vi "SEEK_Common_Socket_Cmd_Sub_VI.vi"(4 "Time Delay":dbl=10.0, 6 "Common Socket Error in":errorcluster, 7 "Response ID 1":u8, 8 "Operation Message Length 1":i32, 9 "Operation Message ID 1":i32, 11 "connection ID":refnum<k5>) -> (0 "Status":string="Horn Scan Success", 1 "error out":errorcluster, 3 "connection ID":refnum<k5>)   [LabVIEW 2017]
panel:
  out "Response from SC":string
  out "Response from SC":u8
  out "Data written to SC":i32
  # "INPUT"
  # "OUTPUT"
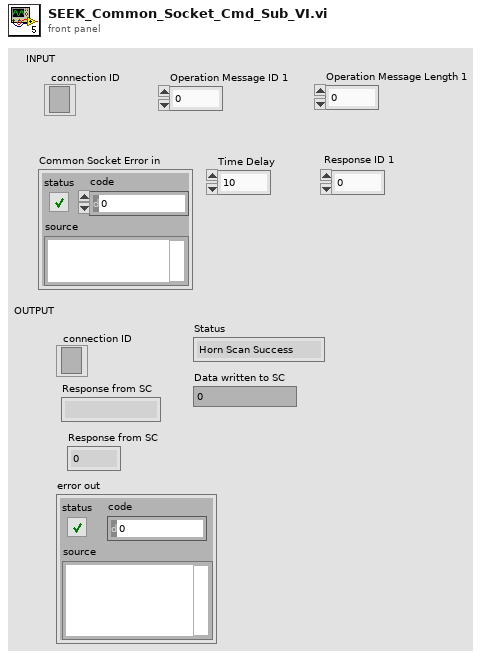
[diagram p1: front panel]
types:
  T1 = enum16{"big-endian, network order", "native, host order", "little-endian"}
  T2 = cluster{"Operation Message Length 1":i32, "Operation Message ID 1":i32}
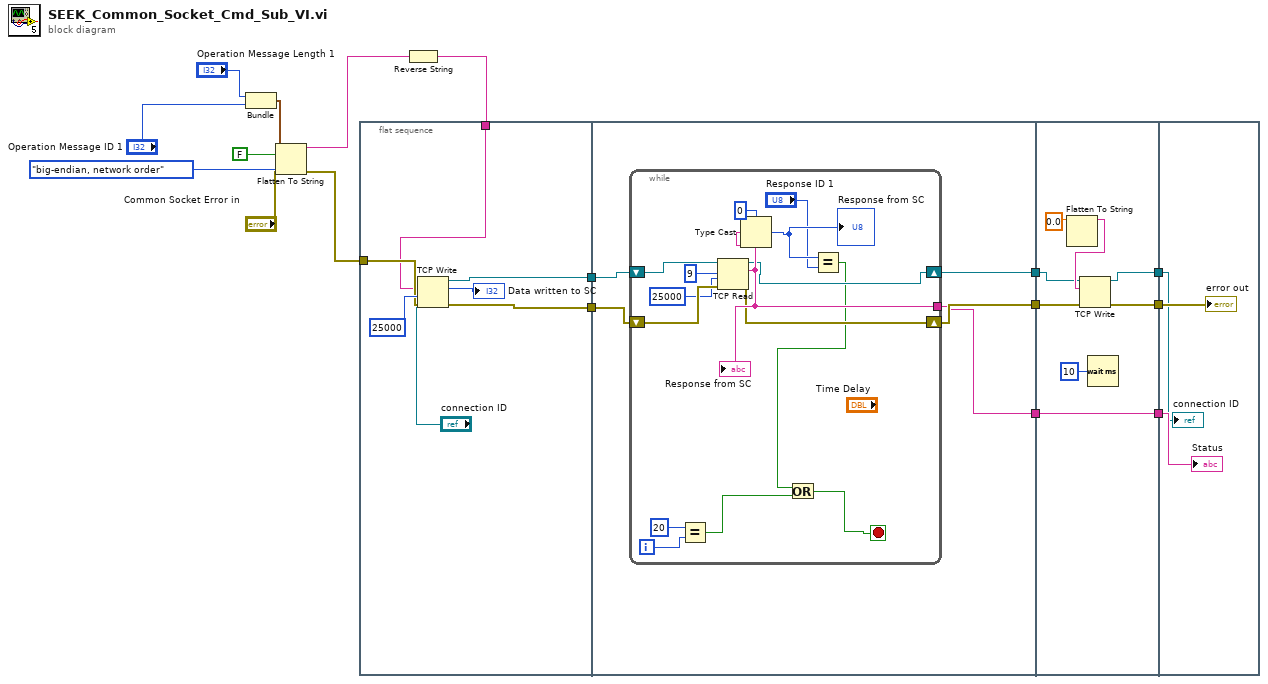
[diagram p0: block diagram]
diagram:
  n1 = Bundle("Operation Message Length 1"="Operation Message Length 1", "Operation Message ID 1"="Operation Message ID 1") -> (w11:T2)  [unwired: 1 in]
  n2 = Flatten To String(anything=w11, prepend array or string size? (T)=FALSE, byte order (0:big-endian, network order)=T1."big-endian, network order", error in (no error)="Common Socket Error in") -> (data string=w13:string, error out=w14:errorcluster)  [unwired: 1 out]
  n3 = flat-sequence {
    tunnel: [w22] -> w2
    tunnel: [w21] -> w1
    tunnel: w14 -> [w20]
    tunnel: w3 -> [w19]
    tunnel: [w29] -> w8
    tunnel: [w28] -> w6
    tunnel: [w27] -> w4
    tunnel: w2 -> [w26]
    tunnel: w1 -> [w25]
    tunnel: [w45] -> w9
    tunnel: w8 -> [w47]
    tunnel: [w52] -> w7
    tunnel: w6 -> [w52]
    tunnel: [w46] -> w5
    tunnel: w4 -> [w48]
    tunnel: w9 -> [w55]
    tunnel: w7 -> [w54]
    tunnel: w5 -> [w53]
    frame #0 {
      n4 = TCP Write(connection ID="connection ID", data in=w19, error in (no error)=w20, 9:25000 ("timeout ms (25000)")) -> (connection ID out=w22:refnum<k5>, bytes written=→"Data written to SC":i32, error out=w21:errorcluster)
    }
    frame #1 {
      n5 = while {
        tunnel: [w41] -> w28
        shift-right: [w33] -> w27
        shift-left: w26 -> [w44]
        shift-right: [w34] -> w29
        shift-left: w25 -> [w43]
        i -> [w37]
        stop <- w30 stop-if-true
        n6 = Equal?(x=20, y=w37) -> (x = y?=w31:bool)
        n7 = TCP Read(connection ID=w44, bytes to read=9, error in (no error)=w43, 9:25000 ("timeout ms (25000)")) -> (connection ID out=w33:refnum<k5>, data out=w41:string, error out=w34:errorcluster)  [unwired: 1 in]
        "Response from SC" <- w41
        n8 = Type Cast(type=u8 0, x=w41) -> (*(type *) &x=w39:u8)
        "Response from SC" <- w39
        n9 = Equal?(x=w39, y="Response ID 1") -> (x = y?=w32:bool)
        n10 = Or(x=w32, y=w31) -> (x .or. y?=w30:bool)
      }
    }
    frame #2 {
      n11 = Flatten To String(anything=0.0) -> (data string=w49:string)  [unwired: 3 in, 2 out]
      n12 = TCP Write(connection ID=w48, data in=w49, error in (no error)=w47) -> (connection ID out=w46:refnum<k5>, error out=w45:errorcluster)  [unwired: 1 in, 1 out]
      n13 = Wait (ms)(milliseconds to wait=u32 10) -> ()  [unwired: 1 out]
    }
    frame #3 {
      "error out" <- w55
      "connection ID" <- w53
      "Status" <- w54
    }
  }
  n14 = Reverse String(1:w13) -> (0:w3:string)
